vi "U32_to_SGL.vi"(4 "U32":u32) -> (1 "SGL":sgl)   [LabVIEW 2017]
doc: "FPGA Casts <b>U32</b> to the data type <b>SGL</b>"
uses:
  <vilib>/rvi/IPIntegrationNode/IPINode_Typedef/niFpgaIPINodeSupportedFamilies.ctl
  <vilib>/rvi/IPIntegrationNode/IPINode_Utilities/niFpgaIPINodeSimCore.vi
  <vilib>/rvi/IPIntegrationNode/IPINode_Xnode/niFpgaIPINode.xnode
  <vilib>/NI/PowerElectronicsControl/ScaleAndLimit/Core/FPGA Type Cast/typecast_U32_to_SGLSimFiles/xsim.dir/typecast_U32_to_SGL/xsimk03D06ED52BF64DBBA65D3792F583FC56.dll
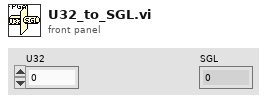
[diagram p1: front panel]
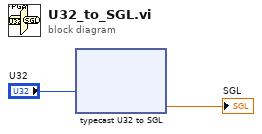
[diagram p0: block diagram]
diagram:
  n1 = xnode ("typecast U32 to SGL")("u32"="U32") -> ("sgl"=→"SGL":sgl)
